vi "Set Library Paths on Child.vi"(7 "SSL-Lib in":refnum<class "SSL-Lib.lvclass">, 8 "error in (no error)":errorcluster, 11 "SSL-Lib in":refnum<class "SSL-Lib.lvclass">) -> (0 "error out":errorcluster, 3 "SSL-Lib out":refnum<class "SSL-Lib.lvclass">)   [LabVIEW 2013, in "OpenSSL Socket.lvlib" / "SSL-Lib.lvclass"]
uses:
  SSL-Lib.lvclass
  SSL-Lib.lvclass/SSL-Lib.ctl
  Read Crypto Library Path.vi
  Read SSL Library Path.vi
  Write Crypto Library Path.vi
  Write SSL Library Path.vi
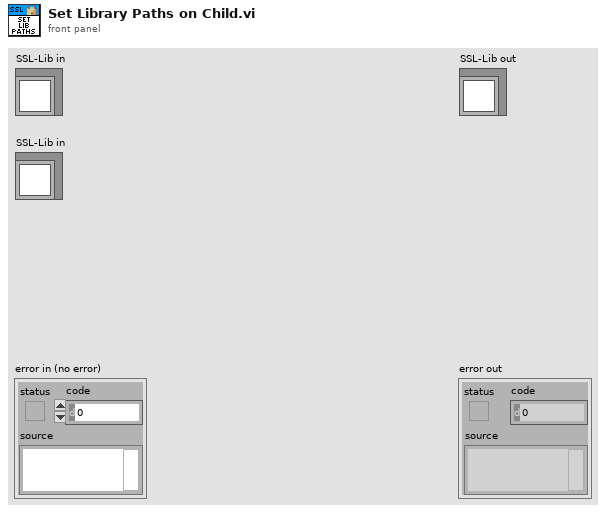
[diagram p1: front panel]
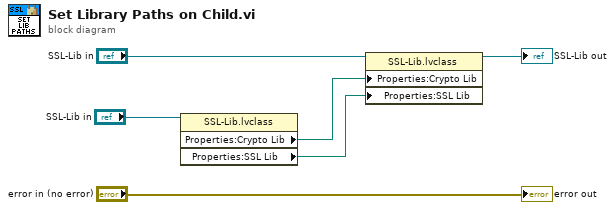
[diagram p0: block diagram]
diagram:
  n1 = property class="SSL-Lib.lvclass"(reference="SSL-Lib in") -> ("Properties:Crypto Lib"=w3:path, "Properties:SSL Lib"=w2:path)  [unwired: 1 in, 2 out]
  n2 = property class="SSL-Lib.lvclass"(reference="SSL-Lib in", "Properties:Crypto Lib"=w3, "Properties:SSL Lib"=w2) -> (reference out=→"SSL-Lib out":refnum<class "SSL-Lib.lvclass">)  [unwired: 1 in, 1 out]
  "error out" <- "error in (no error)"
